vi "Actor Core.vi"(8 "error in":errorcluster, 11 "Template in":refnum<class "Template.lvclass">) -> (0 "error out":errorcluster, 3 "Actor out":refnum<class "Actor.lvclass">)   [LabVIEW 2020, in "Template.lvlib" / "Template.lvclass"]
doc: "(<B>Filename</B>: Actor Framework.lvlib:Actor.lvclass:Actor Core.vi)\n\nReceives messages to the actor, reacts to them, and initiates any error handling that may shut the actor down.\n\nDescendant classes may override this VI to append parallel tasks for the actor to complete while it handles messages. Overrides use the Call Parent Class Method node."
uses:
  Template.lvclass
  <vilib>/ActorFramework/Actor/Actor.lvclass
  Template.lvclass/Template.ctl
  acessors/Read Write Data.vi
  <vilib>/Utility/error.llb/Clear Errors.vi
  methods/fire error event.vi
  methods/monitor stop notification.vi
  methods/send data.vi
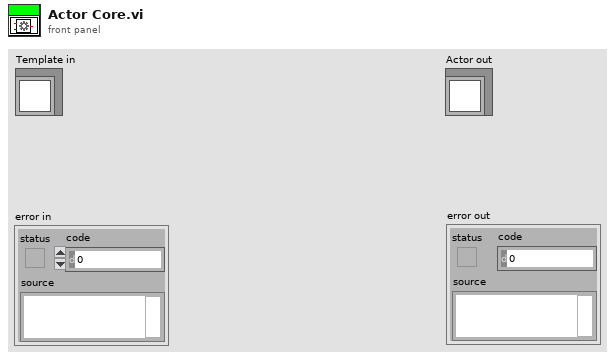
[diagram p1: front panel]
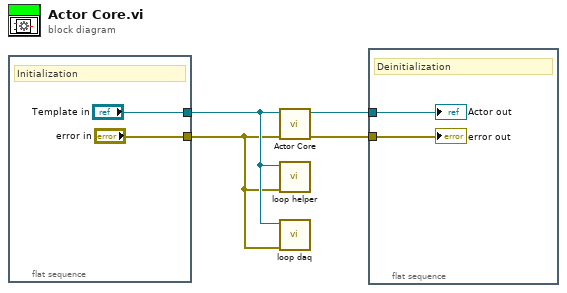
[diagram p0: block diagram]
diagram:
  n1 = flat-sequence {
    tunnel: ["error in"] -> w1
    tunnel: ["Template in"] -> w2
    frame #0 {
      # "Initialization"
    }
  }
  n2 = call-parent "Actor Core.vi"("error in"=w1, "Actor in"=w2) -> ("error out"=w4:errorcluster, "Actor out"=w3:refnum<class "Actor.lvclass">)  [unwired: 8 in]
  n3 = call "loop helper.vi"("error in (no error)"=w1, "Template in"=w2) -> ()  [unwired: 10 in]
  n4 = call "loop daq.vi"("error in (no error)"=w1, "Template in"=w2) -> ()  [unwired: 10 in]
  n5 = flat-sequence {
    tunnel: w4 -> [w8]
    tunnel: w3 -> [w7]
    frame #0 {
      # "Deinitialization"
      "error out" <- w8
      "Actor out" <- w7
    }
  }
